vi "E.vi"(10 "String":string, 11 "format string in":string) -> (3 "format string out":string)   [LabVIEW 2017]
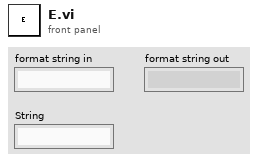
[diagram p1: front panel]
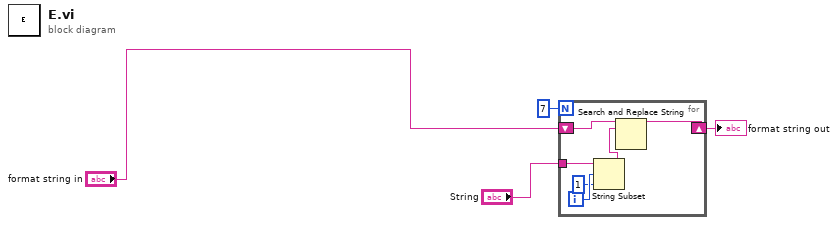
[diagram p0: block diagram]
diagram:
  n1 = for {
    N: 7 -> [_]
    tunnel: "String" -> [w9]
    shift-right: [w5] -> w4
    shift-left: "format string in" -> [w10]
    i -> [w8]
    n2 = String Subset(string=w9, offset (0)=w8, length (rest)=1 ("length (rest)")) -> (substring=w6:string)
    n3 = Search and Replace String(input string=w10, search string=w6) -> (result string=w5:string)  [unwired: 6 in, 3 out]
  }
  "format string out" <- w4
